vi "Tusk.Register.vi"(8 "error in (no error)":errorcluster, 11 "Tusk in":refnum<class "Tusk.lvclass">) -> (0 "error out":errorcluster, 3 "Tusk out":refnum<class "Tusk.lvclass">)   [LabVIEW 2018, in "Application.lvlib" / "Tusk.lvclass"]
uses:
  Tusk.lvclass
  Tusk.lvclass/Tusk.ctl
  Dictionary Class/Dictionary.lvclass/Dictionary.ctl
  ecdc04cd-daca-4470-8ca9-75b19434ba98.vi
  Dictionary Class/VIs/Get Data DVR.vi
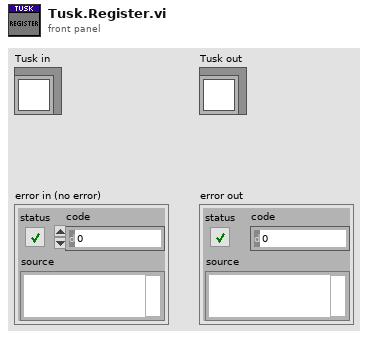
[diagram p1: front panel]
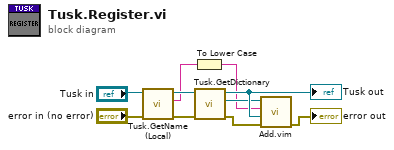
[diagram p0: block diagram]
diagram:
  n1 = call "Tusk.GetName (Local).vi"("error in (no error)"="error in (no error)", "Tusk in"="Tusk in") -> ("error out"=w3:errorcluster, "Name(Local)"=w1:string, "Tusk out"=w4:refnum<class "Tusk.lvclass">)  [unwired: 7 in]
  n2 = To Lower Case(string=w1) -> (all lower case string=w6:string)
  n3 = call "Tusk.GetDictionary.vi"("error in (no error)"=w3, "Tusk in"=w4) -> ("error out"=w8:errorcluster, "Dictionary"=w7:refnum<class "Dictionary.lvclass">, "Tusk out"=w9:refnum<class "Tusk.lvclass">)  [unwired: 7 in]
  "Tusk out" <- w9
  n4 = call "Add.vim"("error in (no error)"=w8, "Value"=w9, "Key"=w6, "Dictionary in"=w7) -> ("error out"=→"error out":errorcluster)  [unwired: 5 in, 2 out]
